vi "CheckSN-Slot2.vi"(6 "Slot":T1, 8 "error out":errorcluster) -> (0 "错误输出":errorcluster, 3 "比对结果":bool, 11 "当前SN":string)   [LabVIEW 2013]
uses:
  SystemCode/SysControl/Slot.ctl
panel:
  out "提示":string
  in  "扫描SN":string
  in  "停止":bool
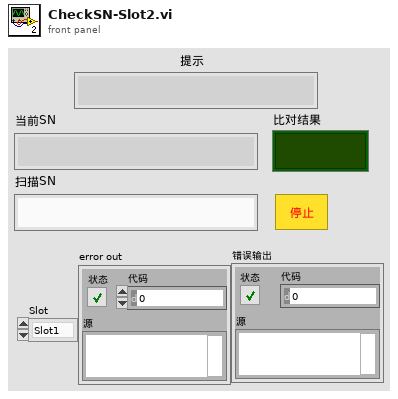
[diagram p1: front panel]
types:
  T1 = typedef "Slot.ctl" = enum16{"Slot1", "Slot2", "Slot3", "Slot4"}
  T2 = typedef "LVRectTypeDef.ctl" = cluster{"Left":i16, "Top":i16, "Right":i16, "Bottom":i16}
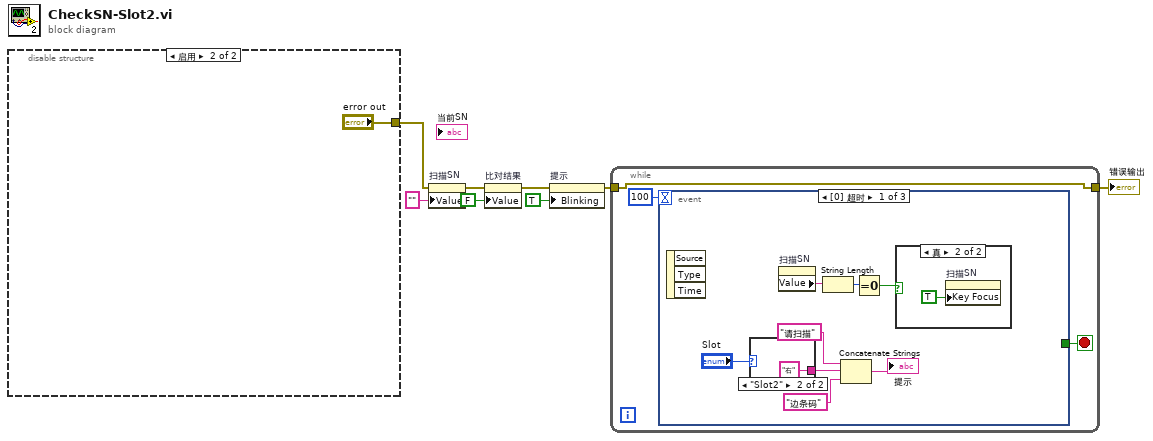
[diagram p0: block diagram]
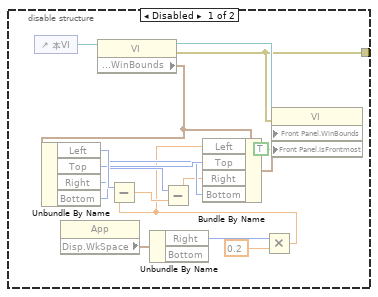
[diagram p2: hidden frame]
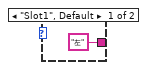
[diagram p3: hidden frame]
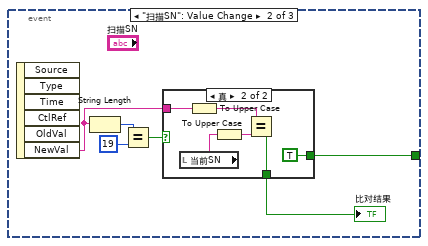
[diagram p5: hidden frame]
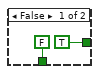
[diagram p6: hidden frame]
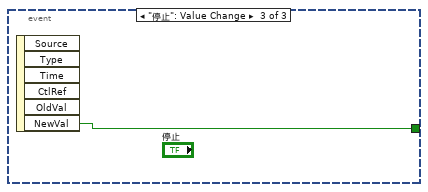
[diagram p7: hidden frame]
diagram:
  n1 = disable-structure shown="启用" {
    disable-tunnel: [w9 "error out"] -> w8
    frame Disabled {
      n2 = control-ref of="本VI"() -> (w24:refnum<vi>)
      n3 = property class="App"() -> ("Disp.WkSpace"=w21:T2)  [unwired: 2 in, 2 out]
      n4 = property class="VI"(reference=w24) -> (reference out=w23:refnum<vi>, error out=w9:errorcluster, "Front Panel.WinBounds"=w19:T2)  [unwired: 1 in]
      n5 = Unbundle By Name(w19) -> ("Left"=w18:i16, "Top"=w17:i16, "Right"=w15:i16, "Bottom"=w16:i16)
      n6 = Unbundle By Name(w21) -> ("Right"=w12:i16)  [unwired: 1 out]
      n7 = Multiply(x=w12, y=0.2) -> (x*y=w11:dbl)
      n8 = Subtract(x=w18, y=w11) -> (x-y=w14:dbl)
      n9 = Subtract(x=w15, y=w14) -> (x-y=w13:dbl)
      n10 = Bundle By Name(cluster=w19, "Left"=w11, "Top"=w17, "Right"=w13, "Bottom"=w16) -> (w22:T2)
      n11 = property class="VI"(reference=w23, error in=w9, "Front Panel.WinBounds"=w22, "Front Panel.IsFrontmost"=TRUE ("前面板窗口:可调整大小")) -> ()  [unwired: 2 out]
    }
    frame Enabled {
    }
  }
  n12 = property on="扫描SN" class="Str"(error in=w8, "Value"="" ("扫描SN")) -> (error out=w3:errorcluster)  [unwired: 1 in, 1 out]
  n13 = property on="比对结果" class="Bool (严格)"(error in=w3, "Value"=FALSE ("比对结果")) -> (error out=w2:errorcluster)  [unwired: 1 in, 1 out]
  n14 = property on="提示" class="Str"(error in=w2, "Blinking"=TRUE ("闪烁")) -> (error out=w6:errorcluster)  [unwired: 1 in, 1 out]
  n15 = while {
    tunnel: w6 -> [w26]
    tunnel: [w26] -> w1
    stop <- w28 stop-if-true
    n16 = event shown="[0] 超时" {
      selector: _ -> [_ _ _]
      dyn-events: _ -> [_ _ _]
      timeout: 100 -> [_ _ _]
      tunnel: [_ w40 w54] -> w28
      event Timeout {
        n17 = event-data() -> ()  [unwired: 1 in, 3 out]
        n18 = case shown="\"Slot2\"" "Slot" {
          tunnel: ["左" ("字符串") "右" ("字符串")] -> w29
          frame "Slot1", Default {
          }
          frame "Slot2" {
          }
        }
        n19 = property on="扫描SN" class="Str"() -> ("Value"=w36:string)  [unwired: 2 in, 2 out]
        n20 = String Length(string=w36) -> (length=w35:i32)
        n21 = Concatenate Strings("请扫描" ("字符串"), w29, "边条码" ("字符串")) -> (→"提示":string)
        n22 = Equal To 0?(x=w35) -> (x = 0?=w34:bool)
        n23 = case shown="真" w34 {
          frame False {
          }
          frame True {
            n24 = property on="扫描SN" class="Str"("Key Focus"=TRUE ("键选中")) -> ()  [unwired: 2 in, 2 out]
          }
        }
      }
      event "扫描SN": Value Change {
        n25 = event-data() -> ("NewVal"=w42:string)  [unwired: 1 in, 5 out]
        n26 = String Length(string=w42) -> (length=w44:i32)
        n27 = Equal?(x=w44, y=19) -> (x = y?=w43:bool)
        n28 = case shown="真" w43 {
          tunnel: w42 -> [_ w51]
          tunnel: [FALSE w49] -> w41
          tunnel: [TRUE TRUE] -> w40
          frame False {
          }
          frame True {
            n29 = local read "当前SN"() -> (w50:string)
            n30 = To Upper Case(1:w51) -> (0:w52:string)
            n31 = To Upper Case(1:w50) -> (0:w53:string)
            n32 = Equal?(x=w52, y=w53) -> (x = y?=w49:bool)
          }
        }
        "比对结果" <- w41
      }
      event "停止": Value Change {
        n33 = event-data() -> ("NewVal"=w54:bool)  [unwired: 1 in, 5 out]
      }
    }
  }
  "错误输出" <- w1
